vi "Encoder Get.vi"(8 "Feet Constant":dbl=1.0, 9 "Tick Constant":dbl=1.0, 10 "Reset":bool, 11 "EncoderDevRef":T2={"DevStatus"={"status"=FALSE, "code"=0, "source"=""}, "EncoderIndex"=enum."Invalid", "CounterIndex"=enum."Invalid", "DistancePerCount"=1.0, "Decoding Type"=enum."4x"}) -> (3 "Encoder Data":T1 {"Ticks" format="%#.6g"})   [LabVIEW 2013]
uses:
  <vilib>/Rock Robotics/WPI/Encoder/WPI_EncoderDevRef.ctl
  <vilib>/Rock Robotics/SystemInterfaces/Encoder/FPGA_EncoderIdx.ctl
  <vilib>/Rock Robotics/SystemInterfaces/Counter/FPGA_CounterCtrSystemIndex.ctl
  <vilib>/Rock Robotics/WPI/Encoder/WPI_EncoderType.ctl
  Single Encoder Data.ctl
  <vilib>/addons/control/pid/pid.llb/PID Control Input Filter (DBL).vi
  <vilib>/addons/control/pid/NI_PID_pid.lvlib
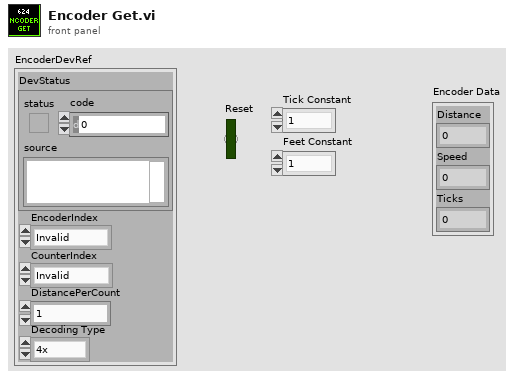
[diagram p1: front panel]
types:
  T1 = typedef "Single Encoder Data.ctl" = cluster{"Distance":dbl, "Speed":dbl, "Ticks":dbl}
  T2 = typedef "WPI_EncoderDevRef.ctl" = cluster{"DevStatus":errorcluster, "EncoderIndex":T3, "CounterIndex":T4, "DistancePerCount":dbl, "Decoding Type":T5}
  T3 = typedef "FPGA_EncoderIdx.ctl" = enum8{"Enc 0", "Enc 1", "Enc 2", "Enc 3", "Invalid"}
  T4 = typedef "FPGA_CounterCtrSystemIndex.ctl" = enum8{"Ctr 0", "Ctr 1", "Ctr 2", "Ctr 3", "Ctr 4", "Ctr 5", "Ctr 6", "Ctr 7", "Invalid"}
  T5 = typedef "WPI_EncoderType.ctl" = enum16{"1x", "2x", "4x"}
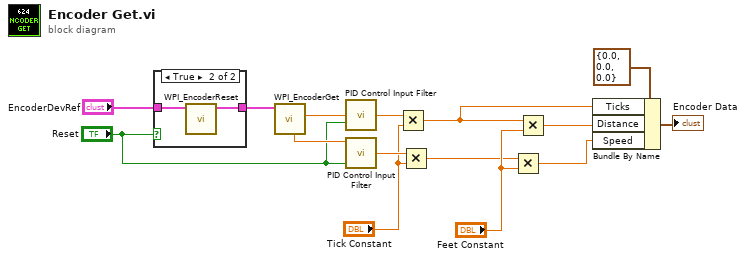
[diagram p0: block diagram]
diagram:
  n1 = case shown="True" "Reset" {
    tunnel: "EncoderDevRef" -> [w16 w18]
    tunnel: [w16 w17] -> w15
    frame False {
    }
    frame True {
      n2 = call <vilib>:"WPI_EncoderReset.vi"("EncoderDevRef"=w18) -> ("EncoderDevRef"=w17:T2)  [unwired: 9 in, 1 out]
    }
  }
  n3 = call <vilib>:"WPI_EncoderGet.vi"("EncoderDevRef"=w15) -> ("Distance"=w13:dbl, "Rate"=w14:dbl)  [unwired: 5 in, 4 out]
  n4 = call-poly <vilib>:"PID Control Input Filter.vi"("reinitialize? (F)"="Reset", "input"=w13) -> ("output"=w5:dbl)  [unwired: 3 in]
  n5 = call-poly <vilib>:"PID Control Input Filter.vi"("reinitialize? (F)"="Reset", "input"=w14) -> ("output"=w7:dbl)  [unwired: 3 in]
  n6 = Multiply(x=w5, y="Tick Constant") -> (x*y=w4:dbl)
  n7 = Multiply(x=w7, y="Tick Constant") -> (x*y=w6:dbl)
  n8 = Multiply(x=w6, y="Feet Constant") -> (x*y=w8:dbl)
  n9 = Multiply(x=w4, y="Feet Constant") -> (x*y=w9:dbl)
  n10 = Bundle By Name(cluster=T1 {"Distance"=0.0, "Speed"=0.0, "Ticks"=0.0} ("Encoder Data"), "Ticks"=w4, "Distance"=w9, "Speed"=w8) -> (→"Encoder Data":T1)
